vi "认识定时循环.vi"() -> ()   [LabVIEW 2018]
uses:
  <vilib>/Platform/TimedLoop/XDataNode/timing_clust.ctl
  <vilib>/Platform/TimedLoop/XDataNode/nitl_modes.ctl
  <vilib>/Platform/TimedLoop/XDataNode/wakeup.ctl
  <vilib>/Platform/TimedLoop/XDataNode/XDataNode.xnode
  <vilib>/Platform/TimedLoop/XDataNode/XDNodeRunTimeDep.lvlib
panel:
  out "延迟完成？":bool
  out "滑动杆":u8(slide) scale=0.0..10.0
  in  "数值":dbl
  out "字符串":string="定时结构使用时间控制程序执行\n包含许多时间函数：定时循环、定时顺序等"
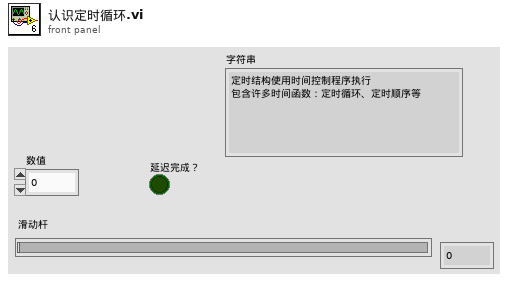
[diagram p1: front panel]
types:
  T1 = typedef "XDNodeRunTimeDep.lvlib/timing_clust.ctl" = cluster{"Expected End [f-1]":u64, "Actual End [f-1]":u64, "Finished Late? [f-1]":bool, "Expected End [i-1]":u64, "Actual End [i-1]":u64, "Finished Late? [i-1]":bool, "Expected Start [i]":u64, "Actual Start [i]":u64, "Expected Start [f]":u64, "Actual Start [f]":u64, "Source Name":string, "Structure Name":string, "Period":i64, "Deadline":i64, "Offset":i64, "Start":i64, "Priority":i32, "Timeout":i32, "Mode":T2, "Wakeup Reason":T3, "Error":errorcluster, "Source Type":string, "Secondary Source Type":string, "Global End Time":u64, "Global Start Time":u64, "Frame Duration":u64, "Iteration Duration":u64, "Assigned CPU":i32, "I/O Scan Engine Mode":u32}
  T2 = typedef "XDNodeRunTimeDep.lvlib/nitl_modes.ctl" = enum32{"No Change", "Process missed periods, maintain original phase", "Discard missed periods, maintain original phase", "Process missed periods, ignore original phase", "Discard missed periods, ignore original phase"}
  T3 = typedef "XDNodeRunTimeDep.lvlib/wakeup.ctl" = enum32{"Normal", "Aborted", "Asynchronous wakeup", "Timing source error", "Timed loop error", "Timeout"}
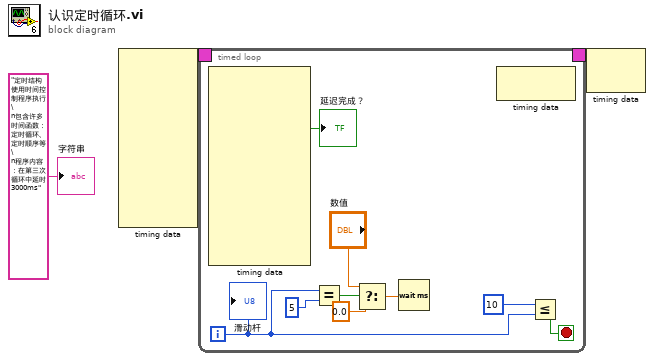
[diagram p0: block diagram]
diagram:
  n1 = node-c288() -> (w2:T1)  [unwired: 10 in]
  n2 = timed-loop {
    timing: w2 -> [_]
    timing-out: [_] -> w1
    i -> [w5]
    stop <- w11 stop-if-true
    n3 = node-c288() -> (→"延迟完成？":bool)  [unwired: 1 in, 11 out]
    n4 = Equal?(x=w5, y=5 ("x")) -> (x = y?=w9:bool)
    n5 = Select(t="数值", s=w9, f=0.0) -> (s? t:f=w6:dbl)
    n6 = Wait (ms)(milliseconds to wait=w6) -> ()  [unwired: 1 out]
    n7 = node-c288() -> ()  [unwired: 1 in, 1 out]
    n8 = Less Or Equal?(x=10, y=w5) -> (x <= y?=w11:bool)
    "滑动杆" <- w5
  }
  n9 = node-c288(w1) -> ()  [unwired: 1 out]
  "字符串" <- "定时结构使用时间控制程序执行\n包含许多时间函数：定时循环、定时顺序等\n程序内容：在第三次循环中延时3000ms"
